vi "ArmSolenoid.vi"(0 "EncoderDistance":dbl) -> ()   [LabVIEW 2018]
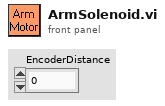
[diagram p1: front panel]
types:
  T1 = typedef "WPI_MotorControlDeviceRef.ctl" = cluster{"DeviceStatus":errorcluster, "Type":T2, "PWM":cluster{"PWM Channel":T3, "DeadBand":T4}, "CAN":cluster{"Device Number":u8, "SetOutput VI Ref":variant, "GetOutput VI Ref":variant, "Enable VI Ref":variant, "Disable VI Ref":variant, "Data":variant}, "Invert":bool, "DIO PWM":cluster{"PWM \"Enable\" Channel":T3, "DIOChannel":T5, "PWM Rate":dbl}}
  T2 = typedef "WPI_MotorControlType.ctl" = enum16{"PWM", "CAN", "DIO PWM"}
  T3 = typedef "FPGA_DIOPWMChannel.ctl" = enum8{"PWM 0", "PWM 1", "PWM 2", "PWM 3", "PWM 4", "PWM 5", "PWM 6", "PWM 7", "PWM 8", "PWM 9", "PWM MXP 0", "PWM MXP 1", "PWM MXP 2", "PWM MXP 3", "PWM MXP 4", "PWM MXP 5", "PWM MXP 6", "PWM MXP 7", "PWM MXP 8", "PWM MXP 9", "Invalid"}
  T4 = typedef "WPI_PWMDeadband.ctl" = cluster{"Name":string, "maxPositivePwm":i32, "minPositivePwm":i32, "centerPwm":i32, "maxNegativePwm":i32, "minNegativePwm":i32, "angularRange":u16}
  T5 = typedef "FPGA_DIOChannel.ctl" = enum8{"DIO 0", "DIO 1", "DIO 2", "DIO 3", "DIO 4", "DIO 5", "DIO 6", "DIO 7", "DIO 8", "DIO 9", "DIO MXP 0", "DIO MXP 1", "DIO MXP 2", "DIO MXP 3", "DIO MXP 4", "DIO MXP 5", "DIO MXP 6", "DIO MXP 7", "DIO MXP 8", "DIO MXP 9", "DIO MXP 10", "DIO MXP 11", "DIO MXP 12", "DIO MXP 13", "DIO MXP 14", "DIO MXP 15", "SPI Port CS1", "SPI Port CS2", "SPI Port CS3", "SPI Port MISO", "SPI Port MOSI", "Invalid"}
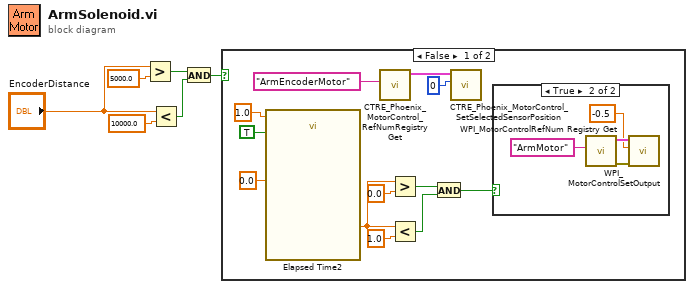
[diagram p0: block diagram]
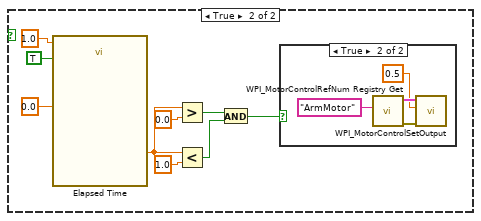
[diagram p3: hidden frame]
diagram:
  n1 = Greater?(x="EncoderDistance", y=5000.0) -> (0:w5:bool)
  n2 = Less?(x="EncoderDistance", y=10000.0) -> (x < y?=w4:bool)
  n3 = And(x=w5, y=w4) -> (x .and. y?=w6:bool)
  n4 = case shown="False" w6 {
    frame False {
      n5 = call "Elapsed Time2"("Time Target (s)"=1.0, "Reset"=TRUE, "Set Start Time (s)"=0.0) -> ("Elapsed Time (s)"=w10:dbl)  [unwired: 9 in, 7 out]
      n6 = call <vilib>:"CTRE_Phoenix_MotorControl_RefNumRegistryGet.vi"("refnum name"="ArmEncoderMotor") -> ("PhoenixMotorControlDevRef"=w18:T1)  [unwired: 9 in, 1 out]
      n7 = Greater?(x=w10, y=0.0) -> (0:w14:bool)
      n8 = Less?(x=w10, y=1.0) -> (x < y?=w13:bool)
      n9 = And(x=w14, y=w13) -> (x .and. y?=w15:bool)
      n10 = call <vilib>:"CTRE_Phoenix_MotorControl_SetSelectedSensorPosition.vi"("New Sensor Position"=0, "PhoenixMotorControlDevRef"=w18) -> ()  [unwired: 8 in, 2 out]
      n11 = case shown="True" w15 {
        frame False {
        }
        frame True {
          n12 = call <vilib>:"WPI_MotorControlRefNum Registry Get.vi"("refnum name"="ArmMotor") -> ("error out"=w21:errorcluster, "MotorControlDevRef"=w22:T1)  [unwired: 9 in]
          n13 = call <vilib>:"WPI_MotorControlSetOutput.vi"("error in (no error)"=w21, "Output"=-0.5, "MotorControlDevRef"=w22) -> ()  [unwired: 6 in, 3 out]
        }
      }
    }
    frame True {
      n14 = call "Elapsed Time"("Time Target (s)"=1.0, "Reset"=TRUE ("Auto Reset"), "Set Start Time (s)"=0.0) -> ("Elapsed Time (s)"=w27:dbl)  [unwired: 9 in, 7 out]
      n15 = Greater?(x=w27, y=0.0) -> (0:w30:bool)
      n16 = Less?(x=w27, y=1.0) -> (x < y?=w31:bool)
      n17 = And(x=w30, y=w31) -> (x .and. y?=w29:bool)
      n18 = case shown="True" w29 {
        frame False {
        }
        frame True {
          n19 = call <vilib>:"WPI_MotorControlRefNum Registry Get.vi"("refnum name"="ArmMotor") -> ("error out"=w34:errorcluster, "MotorControlDevRef"=w35:T1)  [unwired: 9 in]
          n20 = call <vilib>:"WPI_MotorControlSetOutput.vi"("error in (no error)"=w34, "Output"=0.5, "MotorControlDevRef"=w35) -> ()  [unwired: 6 in, 3 out]
        }
      }
    }
  }
